vi "Subvi_Online_SVM_분석기_woF4.vi"(0 "rate":dbl=500.0 caption="Rate" format="%0.2f", 1 "samples per channel":i32=25, 2 "DIscard Channel Info":i32[](array[numeric]), 4 "Brain_data_source":dbl[][](array[numeric]) caption="EEG_Raw_Data" format="%0.3f", 5 "Target_Flash_Order":i64[][](array[numeric]), 6 "Value 2":T1 caption="Value", 7 "svm_model_file":string, 8 "Matrix 2":T1 caption="Matrix", 10 "Target":path, 12 "Nontarget":path) -> (13 "EPR_발생_total":i16[](array[numeric]), 14 "output-0~8":i32, 18 "decision":dbl[](array[numeric]), 19 "ERP_Parameters":dbl[][](array[numeric]))   [LabVIEW 2014]
uses:
  <vilib>/Analysis/Matrix/Datatypes/RealMatrix.ctl
  <vilib>/Analysis/3filter.llb/Filter Passband Type.ctl
  <vilib>/Analysis/baseanly.llb/Mean (DBL).vi
  <vilib>/Analysis/3filter.llb/Butterworth Filter (DBL).vi
  <vilib>/Utility/file.llb/Read From Spreadsheet File (DBL).vi
  <vilib>/Analysis/Matrix/Numeric/Conversions/Array To Matrix - RA.vi
  <vilib>/Analysis/Matrix/Numeric/Multiply/Multiply - RM,RM.vi
  <vilib>/Analysis/Matrix/Numeric/Subtract/Subtract - RM,RM.vi
  <vilib>/Analysis/Matrix/Numeric/Conversions/Matrix To Array - RM.vi
  <vilib>/Analysis/NI_AALBase.lvlib
  <vilib>/Analysis/Matrix/NI_Matrix.lvlib
panel:
  out "전치된 배열":dbl[][](array[numeric])
  out "#channel":i32
  out "#sti 6":i32
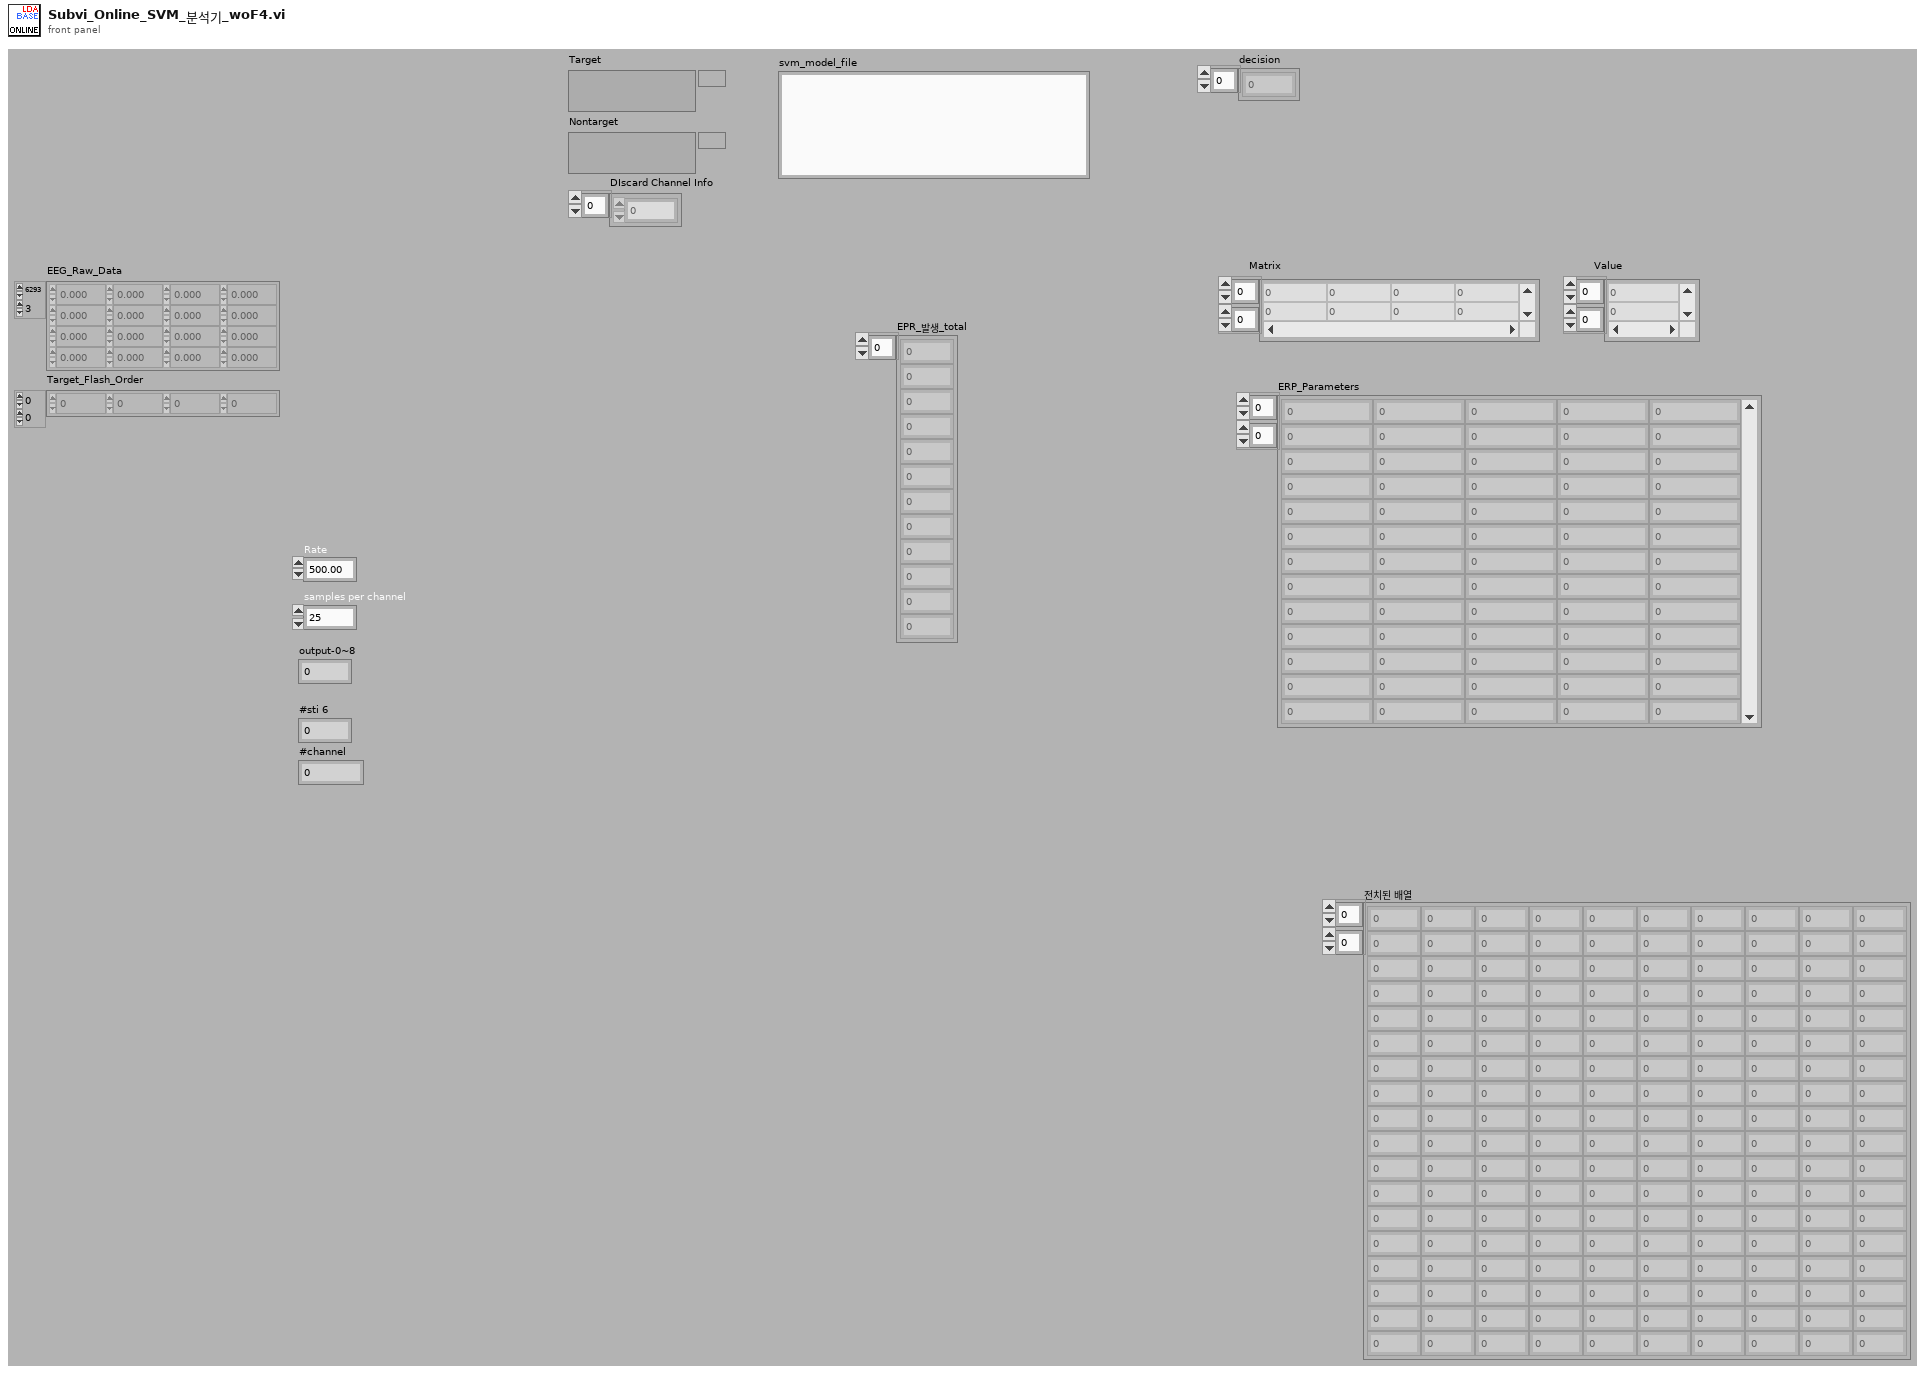
[diagram p1: front panel]
types:
  T1 = typedef "NI_Matrix.lvlib/RealMatrix.ctl" = dbl[][]
  T2 = typedef "NI_AALBase.lvlib/Filter Passband Type.ctl" = enum32{"Lowpass", "Highpass", "Bandpass", "Bandstop"}
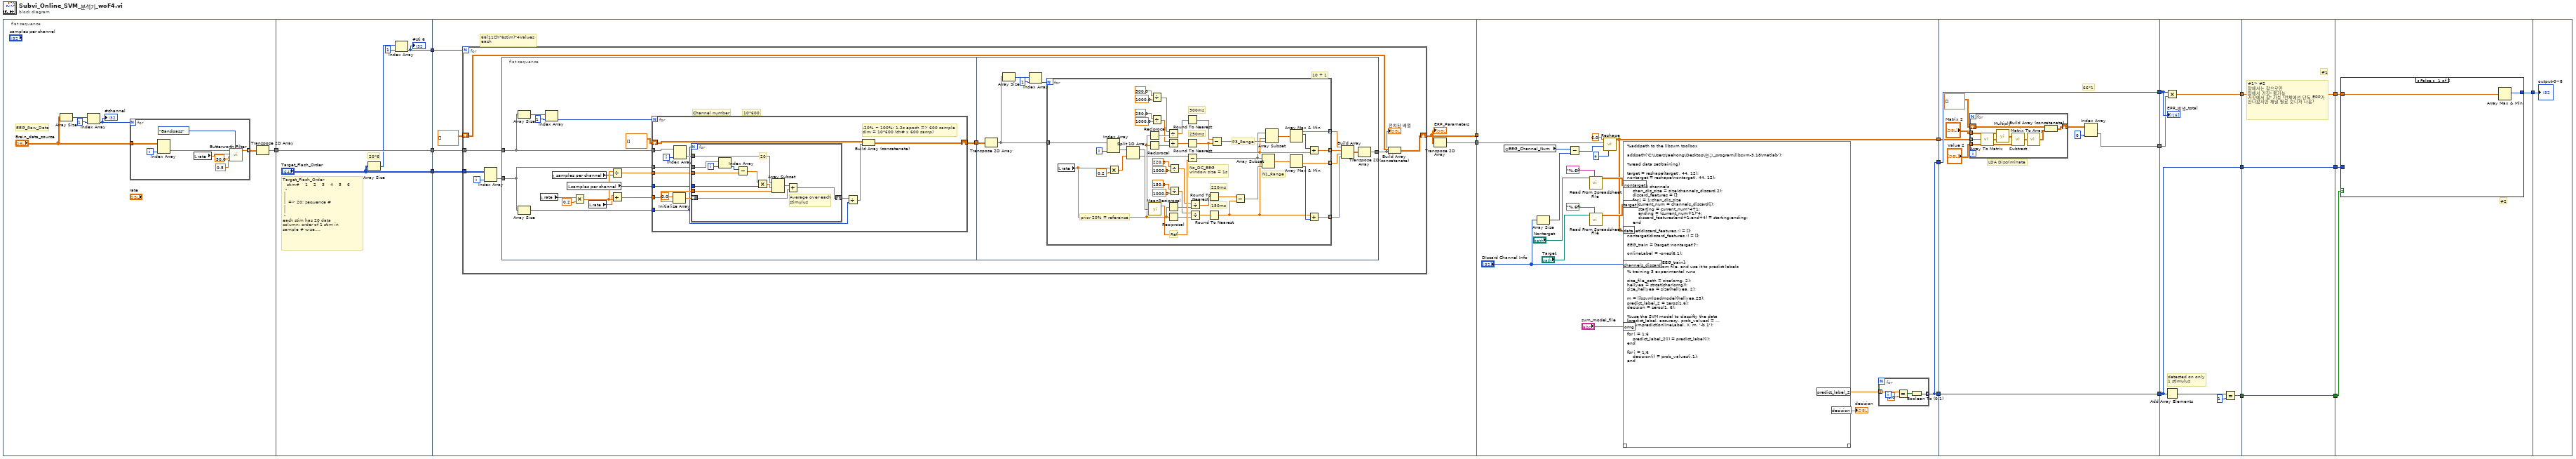
[diagram p0: block diagram]
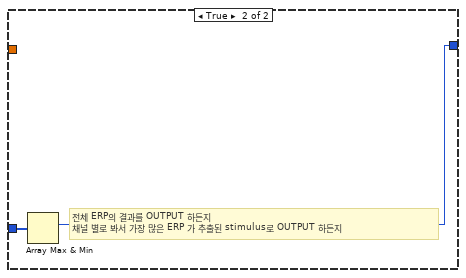
[diagram p2: hidden frame]
diagram:
  n1 = flat-sequence {
    tunnel: [w21] -> w19
    tunnel: [w38] -> w18
    tunnel: ["Target_Flash_Order"] -> w17
    tunnel: w19 -> [w38]
    tunnel: [w35] -> w16
    tunnel: w18 -> [w44]
    tunnel: w17 -> [w43]
    tunnel: w16 -> [w42]
    tunnel: [w39] -> w15
    tunnel: [w40] -> w14
    tunnel: w15 -> [w161]
    tunnel: w14 -> [_]
    tunnel: [w167] -> w6
    tunnel: [w167] -> w4
    tunnel: [w157] -> w1
    tunnel: w6 -> [w180]
    tunnel: [w180] -> w5
    tunnel: w4 -> [w179]
    tunnel: [w179] -> w3
    tunnel: [w173] -> w2
    tunnel: w1 -> [w172]
    tunnel: w5 -> [w190]
    tunnel: [w194] -> w13
    tunnel: w3 -> [w193]
    tunnel: [w191] -> w10
    tunnel: w2 -> [w192]
    tunnel: [w190] -> w9
    tunnel: w13 -> [w197]
    tunnel: [w199] -> w11
    tunnel: w10 -> [w199]
    tunnel: w9 -> [w198]
    tunnel: [w198] -> w8
    tunnel: [w197] -> w7
    tunnel: [w203] -> w12
    tunnel: w11 -> [w202]
    tunnel: w8 -> [w200]
    tunnel: w7 -> [w201]
    tunnel: w12 -> [w208]
    frame #0 {
      # "EEG_Raw_Data"
      n2 = Array Size(array="Brain_data_source") -> (size(s)=w22:i32[])
      n3 = Index Array(array=w22, index=1) -> (element=w24:i32)
      "#channel" <- w24
      n4 = for {
        N: w24 -> [_]
        tunnel: "Brain_data_source" -> [w33]
        tunnel: [w29] -> w25 mode=indexing
        i -> [w32]
        n5 = Index Array(array=w33, index (col)=w32) -> (element=w31:dbl[])  [unwired: 1 in]
        n6 = local read "rate"() -> (w26:dbl)
        n7 = call-poly <vilib>:"Butterworth Filter.vi"("filter type"=Filter_Passband_Type."Bandpass", "low cutoff freq: fl"=0.5, "high cutoff freq: fh"=30.0, "sampling freq: fs"=w26, "X"=w31) -> ("Filtered X"=w29:dbl[])  [unwired: 3 in, 1 out]
      }
      n8 = Transpose 2D Array(2D array=w25) -> (transposed array=w21:dbl[][])
    }
    frame #1 {
      # "Target_Flash_Order\n   stim#    1    2    3    4    5    6    \n  -\n |\n |\n |  => 20: sequence # \n |\n |\n -\neach stim has 20 data\ncolumn: order of 1 stim in \nsample # wise...."
      # "20*6"
      n9 = Array Size(array="Target_Flash_Order") -> (size(s)=w37:i32[])
      n10 = Index Array(array=w37, index=1 ("인덱스")) -> (element=w35:i32)
      "#sti 6" <- w35
    }
    frame #2 {
      # "66(11Ch*6stim)*4Values\neach"
      n11 = for {
        N: w42 -> [_]
        tunnel: w44 -> [w51]
        tunnel: w43 -> [w50]
        shift-right: [w47] -> w40
        shift-left: dbl[][] [] -> [w46]
        i -> [w49]
        n12 = Index Array(array=w50, index (col)=w49) -> (element=w48:i64[])  [unwired: 1 in]
        n13 = flat-sequence {
          tunnel: w51 -> [w55]
          tunnel: w48 -> [w54]
          tunnel: [w53] -> w52
          tunnel: w52 -> [w99]
          tunnel: [w95] -> w45
          frame #0 {
            # "10*600"
            # "Channel number"
            n14 = Array Size(array=w55) -> (size(s)=w58:i32[])
            n15 = Array Size(array=w54) -> (size(s)=w57:i32)
            n16 = local read "rate"() -> (w64:dbl)
            n17 = Index Array(array=w58, index=1) -> (element=w60:i32)
            n18 = local read "samples per channel"() -> (w62:i32)
            n19 = local read "samples per channel"() -> (w61:i32)
            n20 = Multiply(x=w64, y=0.2) -> (x*y=w68:dbl)
            n21 = local read "rate"() -> (w66:dbl)
            n22 = Divide(x=w68, y=w62) -> (x/y=w65:dbl)
            n23 = Add(x=w66, y=w68) -> (x+y=w67:dbl)
            n24 = for {
              N: w60 -> [_]
              tunnel: w61 -> [w69]
              tunnel: w67 -> [w80]
              shift-right: [w73] -> w53
              shift-left: dbl[][] [] -> [w75]
              tunnel: w57 -> [w74]
              tunnel: w55 -> [w72]
              tunnel: w54 -> [w71]
              tunnel: w65 -> [w70]
              i -> [w82]
              # "-20% ~ 100%: 1.2s epoch => 600 sample\ndim = 10*600 (ch# x 600 samp)"
              n25 = Initialize Array(0.0 ("element"), w80) -> (w79:dbl[])
              n26 = Index Array(array=w72, index (col)=w82) -> (element=w81:dbl[])  [unwired: 1 in]
              n27 = for {
                N: w74 -> [_]
                tunnel: w81 -> [w94]
                shift-right: [w91] -> w77
                shift-left: w79 -> [w92]
                tunnel: w80 -> [w90]
                tunnel: w71 -> [w88]
                tunnel: w70 -> [w86]
                tunnel: w69 -> [w84]
                i -> [w89]
                # "Average over each\nstimulus"
                # "20"
                n28 = Index Array(array=w88, index=w89) -> (element=w87:i64)
                n29 = Subtract(x=w87, y=w86) -> (x-y=w85:dbl)
                n30 = Multiply(x=w85, y=w84) -> (x*y=w83:dbl)
                n31 = Array Subset(array=w94, index=w83, length=w90) -> (w93:dbl[])
                n32 = Add(x=w93, y=w92) -> (x+y=w91:dbl[])
              }
              n33 = Divide(x=w77, y=w74) -> (x/y=w76:dbl[])
              n34 = Build Array (concatenate)(w75, w76) -> (w73:dbl[][])
            }
          }
          frame #1 {
            # "10 + 1"
            n35 = Transpose 2D Array(2D array=w99) -> (transposed array=w97:dbl[][])
            n36 = Array Size(array=w97) -> (size(s)=w100:i32[])
            n37 = Index Array(array=w100, index=1) -> (element=w96:i32)
            n38 = for {
              N: w96 -> [_]
              tunnel: w97 -> [w149]
              tunnel: [w144] -> w104 mode=indexing
              tunnel: [w142] -> w103 mode=indexing
              tunnel: [w113] -> w102 mode=indexing
              tunnel: [w139] -> w101 mode=indexing
              i -> [w138]
              # "P3_Range"
              # "N1_Range"
              # "220ms"
              # "150ms"
              # "500ms"
              # "250ms"
              # "No_DC_EEG\nwindow size = 1s"
              # "Ref"
              # "prior 20% = reference"
              n39 = local read "rate"() -> (w120:dbl)
              n40 = Index Array(array=w149, index (col)=w138) -> (element=w141:dbl[])  [unwired: 1 in]
              n41 = Multiply(x=w120, y=0.2) -> (x*y=w147:dbl)
              n42 = Split 1D Array(array=w141, index=w147) -> (first subarray=w146:dbl[], second subarray=w137:dbl[])
              n43 = Reciprocal(x=w120) -> (1/x=w135:dbl)
              n44 = Reciprocal(x=w120) -> (1/x=w136:dbl)
              n45 = call-poly <vilib>:"Mean.vi"("X"=w146) -> ("mean"=w145:dbl)  [unwired: 1 out]
              n46 = Divide(x=500.0, y=1000.0) -> (x/y=w131:dbl)
              n47 = Divide(x=250.0, y=1000.0) -> (x/y=w132:dbl)
              n48 = Divide(x=w131, y=w135) -> (x/y=w118:dbl)
              n49 = Divide(x=w132, y=w136) -> (x/y=w119:dbl)
              n50 = Reciprocal(x=w120) -> (1/x=w133:dbl)
              n51 = Reciprocal(x=w120) -> (1/x=w134:dbl)
              n52 = Divide(x=220.0, y=1000.0) -> (x/y=w129:dbl)
              n53 = Divide(x=150.0, y=1000.0) -> (x/y=w130:dbl)
              n54 = Round To Nearest(number=w118) -> (nearest integer value=w115:dbl)
              n55 = Round To Nearest(number=w119) -> (nearest integer value=w109:dbl)
              n56 = Subtract(x=w137, y=w145) -> (x-y=w106:dbl[])
              n57 = Divide(x=w129, y=w133) -> (x/y=w116:dbl)
              n58 = Divide(x=w130, y=w134) -> (x/y=w117:dbl)
              n59 = Round To Nearest(number=w116) -> (nearest integer value=w114:dbl)
              n60 = Round To Nearest(number=w117) -> (nearest integer value=w111:dbl)
              n61 = Subtract(x=w115, y=w109) -> (x-y=w110:dbl)
              n62 = Subtract(x=w114, y=w111) -> (x-y=w112:dbl)
              n63 = Array Subset(array=w106, index=w111, length=w112) -> (w107:dbl[])
              n64 = Array Subset(array=w106, index=w109, length=w110) -> (w108:dbl[])
              n65 = Array Max & Min(array=w108) -> (max value=w144:dbl, max index (indices)=w143:i32)  [unwired: 2 out]
              n66 = Array Max & Min(array=w107) -> (min value=w113:dbl, min index (indices)=w140:i32)  [unwired: 2 out]
              n67 = Add(x=w143, y=w109) -> (x+y=w142:dbl)
              n68 = Add(x=w111, y=w140) -> (x+y=w139:dbl)
            }
            n69 = Build Array(w104, w103, w102, w101) -> (w98:dbl[][])
            n70 = Transpose 2D Array(2D array=w98) -> (transposed array=w95:dbl[][])
          }
        }
        n71 = Build Array (concatenate)(w46, w45) -> (w47:dbl[][])
        "전치된 배열" <- w45
      }
      "ERP_Parameters" <- w40
      n72 = Transpose 2D Array(2D array=w40) -> (transposed array=w39:dbl[][])
    }
    frame #3 {
      n73 = global read "Control_Panel_정리.vi" "EEG_Channel_Num"() -> (w160:i32)
      n74 = Array Size(array="DIscard Channel Info") -> (size(s)=w151:i32)
      n75 = Subtract(x=w160, y=w151) -> (x-y=w152:i32)
      n76 = call-poly <vilib>:"Read From Spreadsheet File.vi"("format (%.3f)"="%.6f", "file path (dialog if empty)"="Nontarget") -> ("all rows"=w163:dbl[][])  [unwired: 5 in, 4 out]
      n77 = call-poly <vilib>:"Read From Spreadsheet File.vi"("format (%.3f)"="%.6f", "file path (dialog if empty)"="Target") -> ("all rows"=w164:dbl[][])  [unwired: 5 in, 4 out]
      n78 = call "Reshape.vi"("Numeric"=4, "EEG_Channel_Num"=w152, "all rows"=w161, "Numeric 2"=6.0) -> ("Array"=w157:dbl[][])  [unwired: 7 in]
      n79 = script code="%addpath to the libsvm toolbox\n\naddpath('C:\\Users\\Jaehong\\Desktop\\연구_program\\libsvm-3.18\\matlab');\n\n%read data set(training)\n\ntarget = reshape(target', 44, 12);\nnontarget = reshape(nontarget', 44, 12);\n\n% discard channels\n    chan_dis_size = size(channels_discard,2);\n    discard_features = [];\n    for j = 1:chan_dis_size\n        current_num = channels_discard(j);\n        starting = current_num*4+1;\n        ending = (current_num+1)*4;\n        discard_features(end+1:end+4) = starting:ending;\n    end\n\ntarget(discard_features,:) = [];\nnontarget(discard_features,:) = [];\n\nEEG_train = [target';nontarget']';\n\nonlineLabel = -ones(6,1);\n\nX = [(1:6)' data*EEG_train];\n% load model from file, and use it to predict labels\n% training 3 experimental runs\n\nsize_file_path = size(omg, 2);\nhellyea = strcat(char(omg));\nsize_hellyea = size(hellyea, 2);\n\nm = libsvmloadmodel(hellyea,25);\npredict_label_2 = zeros(1,6);\ndecision = zeros(1, 6);\n\n%use the SVM model to classifty the data\n[predict_label, accuracy, prob_values] = ...\n    svmpredict(onlineLabel, X, m, '-b 1');\n\nfor i = 1:6\n    predict_label_2(i) = predict_label(i);\nend\n\nfor i = 1:6\n    decision(i) = prob_values(i,1);\nend"("target"=w164, "nontarget"=w163, "data"=w157, "omg"="svm_model_file", "channels_discard"="DIscard Channel Info") -> ("predict_label_2"=w162:dbl[], "decision"=→"decision":dbl[])  [unwired: 1 in, 1 out]
      n80 = for {
        tunnel: w162 -> [w171] mode=indexing
        tunnel: [w170] -> w167 mode=indexing
        n81 = Equal?(x=w171, y=1.0) -> (x = y?=w168:bool)
        n82 = Boolean To (0,1)(Boolean=w168) -> (0, 1=w170:i16)
      }
    }
    frame #4 {
      # "LDA Discriminate"
      # "66*1"
      n83 = for {
        tunnel: "Matrix 2" -> [w181]
        tunnel: "Value 2" -> [w187]
        shift-right: [w184] -> w176
        shift-left: dbl[][] [] -> [w183]
        tunnel: w172 -> [w182] mode=indexing
        n84 = call-poly <vilib>:"Array To Matrix.vi"("Real 1D Array"=w182) -> ("Real Matrix (Column Vector)"=w186:T1)
        n85 = call-poly <vilib>:"Multiply.vi"("Real Matrix B"=w186, "Real Matrix A"=w181) -> ("A * B"=w189:T1)
        n86 = call-poly <vilib>:"Subtract.vi"("Real Matrix B"=w187, "Real Matrix A"=w189) -> ("A - B"=w188:T1)
        n87 = call-poly <vilib>:"Matrix To Array.vi"("Real Matrix"=w188) -> ("Real 2D Array"=w185:dbl[][])
        n88 = Build Array (concatenate)(w183, w185) -> (w184:dbl[][])
      }
      n89 = Index Array(array=w176, index (col)=0 ("비활성화된 인덱스 (열)")) -> (element=w173:dbl[])  [unwired: 1 in]
    }
    frame #5 {
      # "detected on only\n1 stimulus"
      n90 = Add Array Elements(numeric array=w190) -> (sum=w196:i16)
      n91 = Multiply(x=w193, y=w192) -> (x*y=w191:dbl[])
      n92 = Equal?(x=w196, y=i16 1) -> (x = y?=w194:bool)
      "EPR_발생_total" <- w193
    }
    frame #6 {
      # "#1> #2\n참에서는 참으로만\n참에서 거짓: 불가능\n거짓에서 참: 가능 (전체에선 단독 ERP가 안나왔지만 채널 별로 보니까 나옴)"
      # "#1"
    }
    frame #7 {
      # "#2"
      n93 = case shown="False" w201 {
        tunnel: [w205 w207] -> w203
        tunnel: w202 -> [w204 _]
        tunnel: w200 -> [_ w206]
        frame False {
          n94 = Array Max & Min(array=w204) -> (max index (indices)=w205:i32)  [unwired: 3 out]
        }
        frame True {
          # "전체 ERP의 결과를 OUTPUT 하든지\n채널 별로 봐서 가장 많은 ERP 가 추출된 stimulus로 OUTPUT 하든지"
          n95 = Array Max & Min(array=w206) -> (max index (indices)=w207:i32)  [unwired: 3 out]
        }
      }
    }
    frame #8 {
      "output-0~8" <- w208
    }
  }
